vi "Step Core.vi"(8 "error in (no error)":errorcluster, 11 "DCPower in":refnum<class "DCPower.lvclass">) -> (0 "error out":errorcluster, 3 "DCPower out":refnum<class "DCPower.lvclass">)   [LabVIEW 2018, in "DCPower.lvlib" / "DCPower.lvclass"]
uses:
  DCPower.lvclass
  C:/Sequence Automation/Plugins/Measurement Interface.lvlibp/Measurement Interface.lvclass
  DCPower.lvclass/DCPower.ctl
  Read DC Pins.vi
  Plugins/Measurement Interface.lvlibp/Private Methods/Measurement Name/Read Measurement Name.vi
  Plugins/Measurement Interface.lvlibp/Private Methods/Engine Reference/Read Engine Reference.vi
  Plugins/Measurement Interface.lvlibp/Measurement Interface.lvclass
  Plugins/TestStand API Tools (TSAT).lvlibp/Step Actions/TSAT Step Actions.lvlib
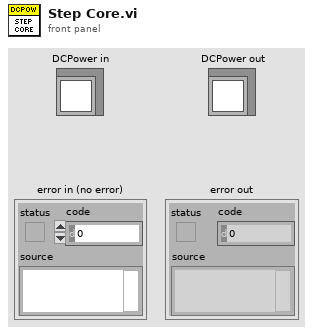
[diagram p1: front panel]
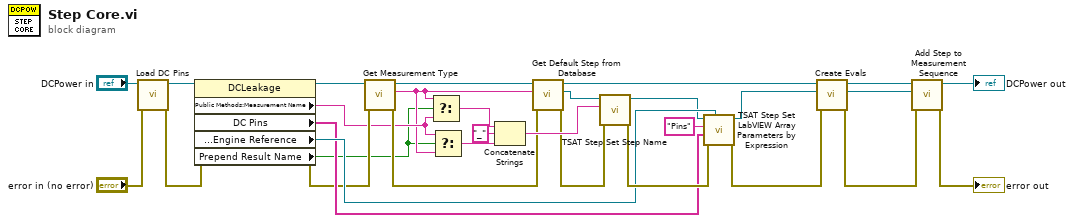
[diagram p0: block diagram]
diagram:
  n1 = call "Load DC Pins.vi"("error in (no error)"="error in (no error)", "DCPower in"="DCPower in") -> ("error out"=w25:errorcluster, "DCPower out"=w23:refnum<class "DCPower.lvclass">)  [unwired: 8 in]
  n2 = property class="DCLeakage"(reference=w23, error in=w25) -> (reference out=w9:refnum<class "DCPower.lvclass">, error out=w7:errorcluster, "Public Methods:Measurement Name"=w3:string, "DC Pins"=w17:string[], "Protected Methods:Engine Reference"=w20:refnum<k7>, "Prepend Result Name"=w1:bool)
  n3 = call-dynamic "Get Measurement Type.vi"("error in (no error)"=w7, "DCPower in"=w9) -> ("error out"=w6:errorcluster, "Measurement Type"=w2:string, "DCPower out"=w8:refnum<class "DCPower.lvclass">)  [unwired: 7 in]
  n4 = Select(t=w2, s=w1, f=w3) -> (s? t:f=w5:string)
  n5 = Select(t=w3, s=w1, f=w2) -> (s? t:f=w4:string)
  n6 = Concatenate Strings(w5, "_" ("string"), w4) -> (w28:string)
  n7 = call "Get Default Step from Database.vi"("error in (no error)"=w6, "Default Step"=w2, "Measurement Interface in"=w8) -> ("error out"=w26:errorcluster, "Cloned Step"=w27:refnum<k7>, "Measurement Interface out"=w15:refnum<class "DCPower.lvclass">)  [unwired: 6 in]
  n8 = call "TSAT Step Set Step Name.vi"("Error In"=w26, "Name"=w28, "Step In"=w27) -> ("Error Out"=w22:errorcluster, "Step Out"=w19:refnum<k7>)  [unwired: 7 in]
  n9 = call "TSAT Step Set LabVIEW Array Parameters by Expression.vi"("Engine In"=w20, "Error In"=w22, "Value Expressions"=w17, "Parameter to Set"="Pins", "Step In"=w19) -> ("Error Out"=w21:errorcluster, "Step Out"=w14:refnum<k7>)  [unwired: 5 in]
  n10 = call-dynamic "Create Evals.vi"("error in (no error)"=w21, "Step In"=w14, "DCPower in"=w15) -> ("error out"=w16:errorcluster, "Step Out"=w10:refnum<k7>, "DCPower out"=w12:refnum<class "DCPower.lvclass">)  [unwired: 6 in]
  n11 = call "Add Step to Measurement Sequence.vi"("error in (no error)"=w16, "Step to Add"=w10, "Measurement Interface in"=w12) -> ("error out"=→"error out":errorcluster, "Measurement Interface out"=→"DCPower out":refnum<class "DCPower.lvclass">)  [unwired: 7 in]
